vi "PlLoN_grabber_recovery_no chart.vi"(7 "Number of Images":u32=1 min=1 step=1, 8 "error in (no error)":errorcluster, 10 "refnum":refnum<file>, 11 "Camera Handle":u32) -> (0 "error out":errorcluster, 1 "DATA":u16[][](array[numeric]), 2 "Number of Images":u32=1 min=1 step=1, 3 "Camera Handle":u32, 4 "x>y?":bool, 5 "refnum out":refnum<file>, 9 "Frame Rate":dbl=1001.0010010010011)   [LabVIEW 2015]
panel:
  out "PyLoN Ready":bool
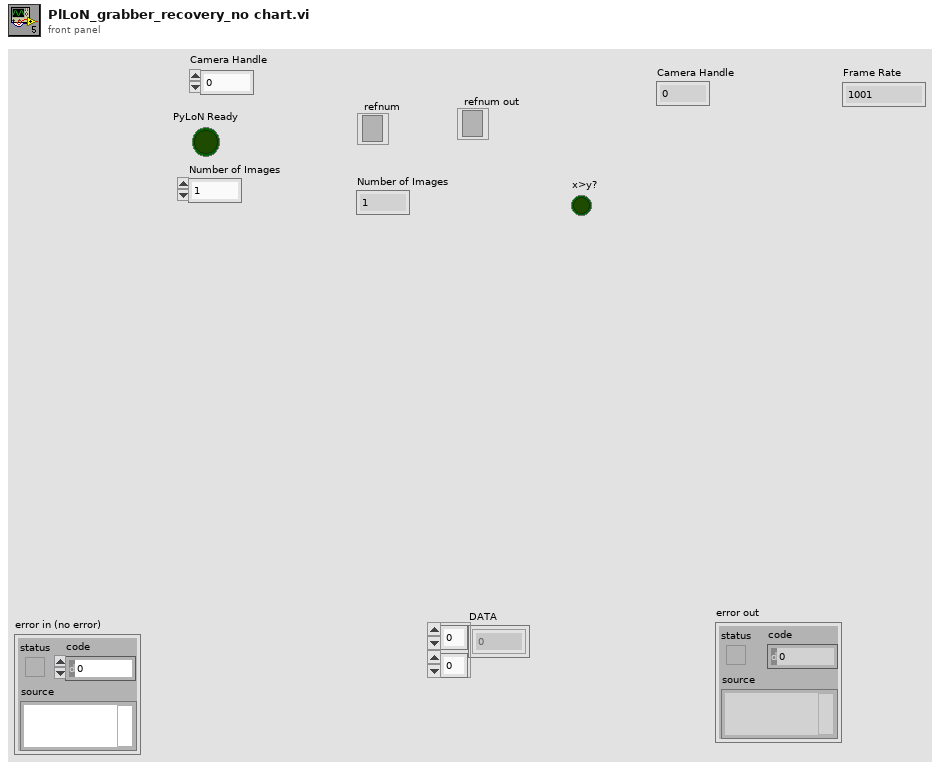
[diagram p1: front panel]
types:
  T1 = cluster{"acquire focus mode":u32, "Exposure Time (s)":dbl, "Number of Images":u32, "Software accumulation":u32}
  T2 = cluster{"Camera Handle":u32, "Pulser Handle":u32, "File Handle":u32, "Display Handle":u32, "Image Handle":u32}
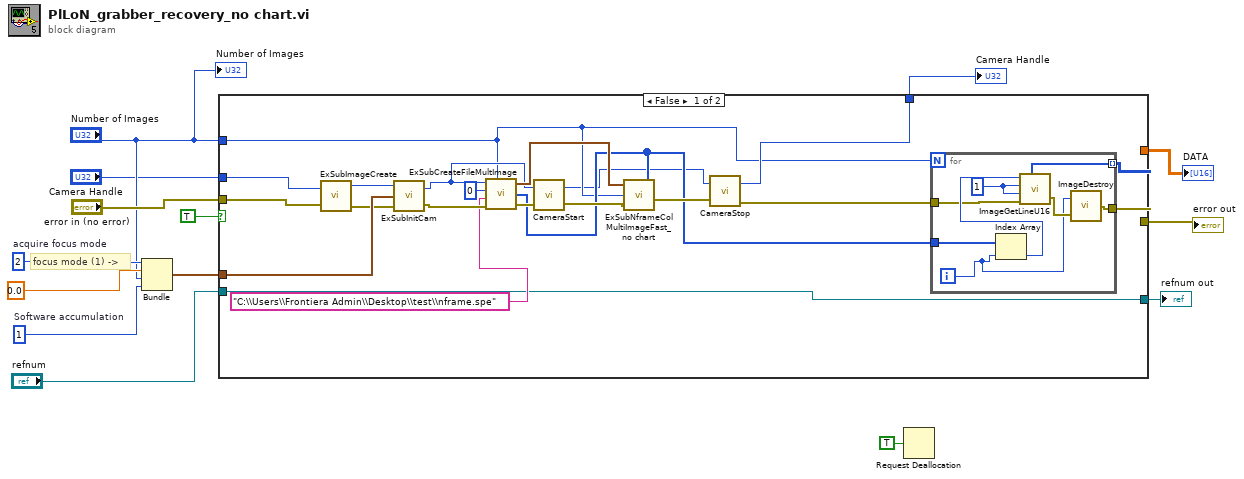
[diagram p0: block diagram]
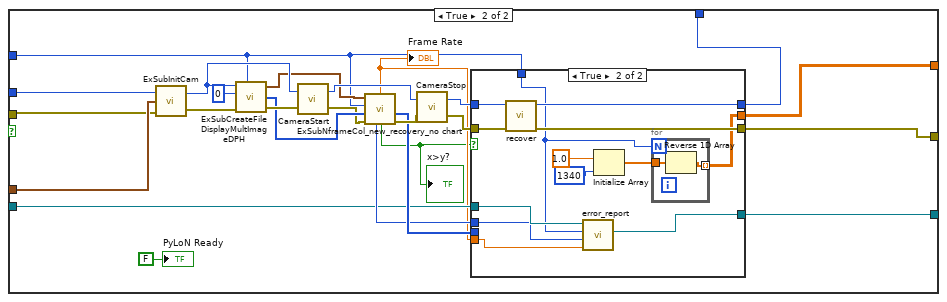
[diagram p2: hidden frame]
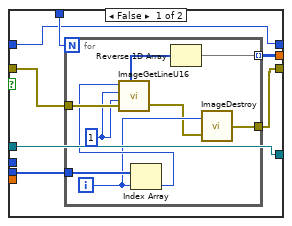
[diagram p3: hidden frame]
diagram:
  w9 = u32 2  # acquire focus mode
  w10 = u32 1  # Software accumulation
  # "focus mode (1) ->"
  n1 = Bundle("acquire focus mode"=w9, "Exposure Time (s)"=0.0, "Number of Images"="Number of Images", "Software accumulation"=w10) -> (w8:T1)  [unwired: 1 in]
  n2 = case shown="False" TRUE {
    tunnel: [w20 w48] -> w4
    tunnel: [w18 w52] -> w14
    tunnel: [w19 w51] -> w13
    tunnel: "Number of Images" -> [w17 w50]
    tunnel: "error in (no error)" -> [w35 w56]
    tunnel: w8 -> [w33 w62]
    tunnel: "Camera Handle" -> [w31 w57]
    tunnel: "refnum" -> [w15 w46]
    tunnel: [w15 w47] -> w2
    frame False {
      n3 = call "ExSubImageCreate.vi"("Camera Handle"=w31, "error in (no error)"=w35) -> ("Camera Handle"=w34:u32, "error out"=w32:errorcluster)  [unwired: 1 out]
      n4 = call "ExSubInitCam.vi"("error in (no error)"=w32, "Camera Information"=w33, "Camera Handle"=w34) -> ("error out"=w30:errorcluster, "Camera Handle"=w24:u32)
      n5 = call "ExSubCreateFileMultImage.vi"("Camera Handle"=w24, "Pulser Handle"=u32 0, "File and Display Name"="C:\\Users\\Frontiera Admin\\Desktop\\test\\nframe.spe", "error in (no error)"=w30, "Number of Images"=w17) -> ("Handles Out"=w25:T2, "Array"=w22:u32[], "error out"=w27:errorcluster)
      n6 = call <userlib>:"CameraStart.vi"("error in"=w27, "Camera Handle"=w24) -> ("error out"=w26:errorcluster, "Camera Handle"=w16:u32)
      n7 = call "ExSubNframeColMultiImageFast_no chart.vi"("Handle Cluster"=w25, "Number of Images"=w17, "error in (no error)"=w26, "image handles"=w22) -> ("error out"=w23:errorcluster)  [unwired: 1 in, 1 out]
      n8 = call <userlib>:"CameraStop.vi"("error in"=w23, "Camera Handle"=w16) -> ("error out"=w21:errorcluster, "Camera Handle"=w18:u32)
      n9 = for {
        N: w17 -> [_]
        tunnel: w22 -> [w43]
        tunnel: w21 -> [w40]
        tunnel: [w39] -> w20 mode=indexing
        tunnel: [w37] -> w19
        i -> [w36]
        w41 = u32 1 ("Y Position")
        n10 = Index Array(array=w43, index=w36) -> (element=w42:u32)
        n11 = call <userlib>:"ImageGetLineU16.vi"("Data Handle"=w42, "Y Position"=w41, "Z Position"=w41, "error in"=w40) -> ("Array u16"=w39:u16[], "error out"=w38:errorcluster)  [unwired: 1 out]
        n12 = call <userlib>:"ImageDestroy.vi"("error in"=w38, "Data handle"=w36) -> ("error out"=w37:errorcluster)
      }
    }
    frame True {
      n13 = call "ExSubInitCam.vi"("error in (no error)"=w56, "Camera Information"=w62, "Camera Handle"=w57) -> ("error out"=w66:errorcluster, "Camera Handle"=w64:u32)
      n14 = call "ExSubCreateFileDisplayMultImageDPH.vi"("Camera Handle"=w64, "Pulser Handle"=u32 0, "error in (no error)"=w66, "Number of Images"=w50) -> ("Handles Out"=w61:T2, "Array"=w60:u32[], "error out"=w65:errorcluster)  [unwired: 1 in]
      n15 = call <userlib>:"CameraStart.vi"("error in"=w65, "Camera Handle"=w64) -> ("error out"=w59:errorcluster, "Camera Handle"=w67:u32)
      n16 = call "ExSubNframeCol_new_recovery_no chart.vi"("error in (no error)"=w59, "image handles"=w60, "Number of Images"=w50, "Handle Cluster 2"=w61) -> ("error out"=w58:errorcluster, "data handles"=w53:u32[], "x > y?"=w44:bool, "Frame Rate"=w45:dbl, "image #"=w49:i32)  [unwired: 2 in, 1 out]
      "Frame Rate" <- w45
      "x>y?" <- w44
      n17 = call <userlib>:"CameraStop.vi"("error in"=w58, "Camera Handle"=w67) -> ("error out"=w55:errorcluster, "Camera Handle"=w54:u32)
      n18 = case shown="True" w44 {
        tunnel: w55 -> [w74 w95]
        tunnel: [w73 w94] -> w51
        tunnel: w54 -> [w70 w97]
        tunnel: [w70 w96] -> w52
        tunnel: w53 -> [w75 _]
        tunnel: w50 -> [w72 w89]
        tunnel: w49 -> [_ w86]
        tunnel: w46 -> [w69 w91]
        tunnel: [w71 w87] -> w48
        tunnel: [w69 w90] -> w47
        tunnel: w45 -> [_ w85]
        frame False {
          n19 = for {
            N: w72 -> [_]
            tunnel: w75 -> [w81]
            tunnel: w74 -> [w84]
            tunnel: [w76] -> w71 mode=indexing
            tunnel: [w78] -> w73
            i -> [w80]
            w83 = u32 1
            n20 = Index Array(array=w81, index=w80) -> (element=w82:u32)
            n21 = call <userlib>:"ImageGetLineU16.vi"("Data Handle"=w82, "Y Position"=w83, "Z Position"=w83, "error in"=w84) -> ("Array u16"=w77:u16[], "error out"=w79:errorcluster)  [unwired: 1 out]
            n22 = Reverse 1D Array(array=w77) -> (reversed array=w76:u16[])
            n23 = call <userlib>:"ImageDestroy.vi"("error in"=w79, "Data handle"=w80) -> ("error out"=w78:errorcluster)
          }
        }
        frame True {
          n24 = call "recover.vi"("error in (no error)"=w95, "Camera Handle"=w97) -> ("error out"=w94:errorcluster, "Camera Handle"=w96:u32)  [unwired: 7 in, 1 out]
          n25 = call "error_report.vi"("_Frame Rate"=w85, "frame #"=w86, "# of frame"=w89, "refnum"=w91) -> ("refnum out"=w90:refnum<file>)  [unwired: 6 in, 1 out]
          n26 = Initialize Array(1.0 ("element"), 1340 ("dimension size")) -> (w88:dbl[])
          n27 = for {
            N: w89 -> [_]
            tunnel: w88 -> [w98]
            tunnel: [w99] -> w87 mode=indexing
            n28 = Reverse 1D Array(array=w98) -> (reversed array=w99:dbl[])
          }
        }
      }
      "PyLoN Ready" <- FALSE ("PyLoN Ready")
    }
  }
  "error out" <- w13
  "DATA" <- w4
  "Camera Handle" <- w14
  "refnum out" <- w2
  n29 = Request Deallocation(TRUE ("flag")) -> ()
  "Number of Images" <- "Number of Images"
